vi "ChoosePlay.vi"(8 "error in (no error)":errorcluster, 9 "currentPlay":refnum<class "Play_v2.lvclass">, 10 "plays":refnum<class "Play_v2.lvclass">[](array[class]), 11 "Playbook_v2 in":refnum<class "Playbook_v2.lvclass">) -> (0 "error out":errorcluster, 2 "newPlay":refnum<class "Play_v2.lvclass">, 3 "Playbook_v2 out":refnum<class "Playbook_v2.lvclass">)   [LabVIEW 2023, in "Playbook_v2.lvclass"]
uses:
  Playbook_v2.lvclass
  NewPlays/Play_v2_class/Play_v2.lvclass
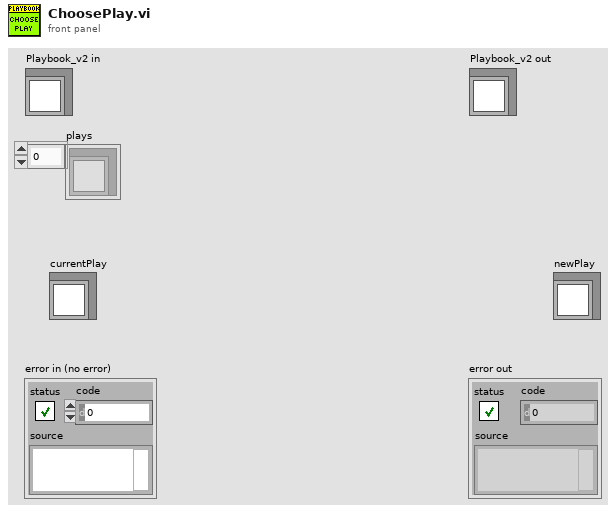
[diagram p1: front panel]
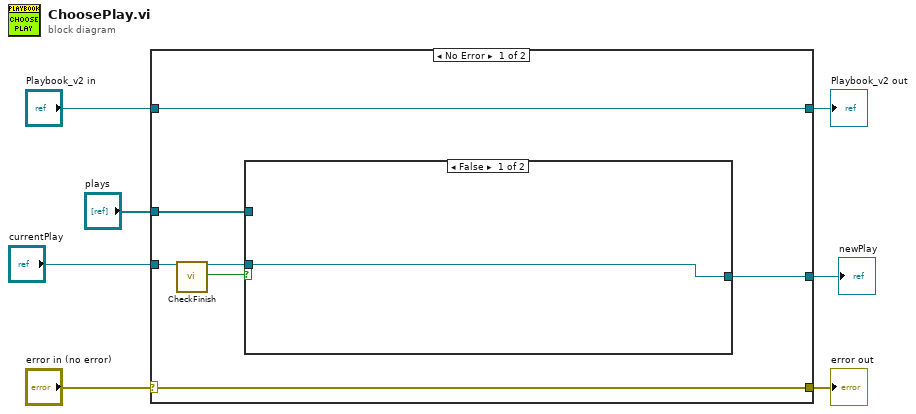
[diagram p0: block diagram]
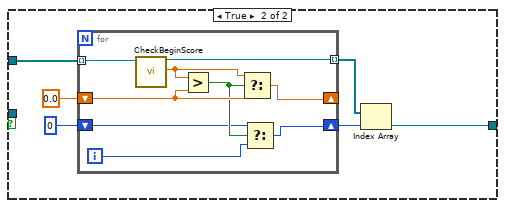
[diagram p2: hidden frame]
diagram:
  n1 = case shown="No Error" "error in (no error)" {
    selector: "error in (no error)" -> [w14 w33]
    tunnel: [w14 w33] -> w6
    tunnel: [w13 w32] -> w4
    tunnel: "Playbook_v2 in" -> [w13 w32]
    tunnel: "currentPlay" -> [w12 w31]
    tunnel: "plays" -> [w10 _]
    tunnel: [w8 w31] -> w1
    frame No Error {
      n2 = call-dynamic "CheckFinish.vi"("object in"=w12) -> ("object out"=w9:refnum<class "Play_v2.lvclass">, "Finish"=w11:bool)  [unwired: 16 in, 1 out]
      n3 = case shown="False" w11 {
        tunnel: w10 -> [_ w21]
        tunnel: [w15 w17] -> w8
        tunnel: w9 -> [w15 _]
        frame False {
        }
        frame True {
          n4 = for {
            tunnel: w21 -> [w22] mode=indexing
            shift-right: [w25] -> w16
            shift-left: 0 -> [w26]
            shift-right: [w28] -> _
            shift-left: 0.0 -> [w29]
            tunnel: [w23] -> w18 mode=indexing
            i -> [w24]
            n5 = call-dynamic "CheckBeginScore.vi"("object in"=w22) -> ("object out"=w23:refnum<class "Play_v2.lvclass">, "score"=w30:dbl)  [unwired: 16 in, 1 out]
            n6 = Greater?(x=w30, y=w29) -> (0:w27:bool)
            n7 = Select(t=w30, s=w27, f=w29) -> (s? t:f=w28:dbl)
            n8 = Select(t=w26, s=w27, f=w24) -> (s? t:f=w25:i32)
          }
          n9 = Index Array(array=w18, index=w16) -> (element=w17:refnum<class "Play_v2.lvclass">)
        }
      }
    }
    frame Error {
    }
  }
  "error out" <- w6
  "Playbook_v2 out" <- w4
  "newPlay" <- w1
